vi "ELVIS III v1.0 Unreserve UART.vi"(8 "error in (no error)":errorcluster, 10 "VISA resource name in":refnum<visa-resource-name>, 11 "myRIO FPGA Ref In":T1) -> (0 "error out":errorcluster)   [LabVIEW 2021]
uses:
  <vilib>/myRIO/Common/Instrument Driver Framework/Utilities/typedefs/Generic FPGA Reference.ctl
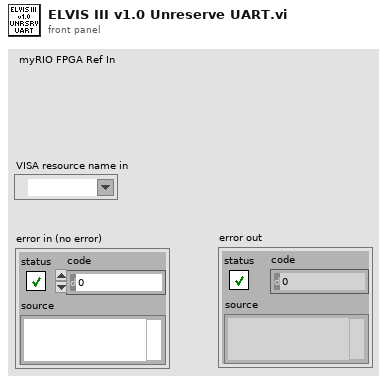
[diagram p1: front panel]
types:
  T1 = typedef "Generic FPGA Reference.ctl" = refnum<k20>
  T2 = typedef "ELVIS III v1.0 Channel Reservation List.ctl" = T3[]
  T3 = typedef "ELVIS III v1.0 Channel Reservation Info.ctl" = cluster{"Channel Name":string, "Connector":T4, "MutexIDs":u32[]}
  T4 = typedef "ELVIS III v1.0 Connector List.ctl" = enum32{"None", "ConnectorA", "ConnectorB"}
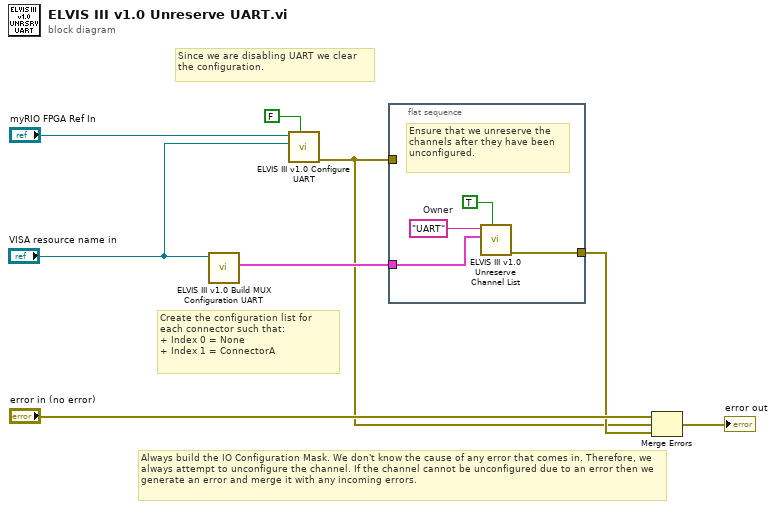
[diagram p0: block diagram]
diagram:
  # "Since we are disabling UART we clear the configuration."
  # "Always build the IO Configuration Mask. We don't know the cause of any error that comes in. Therefore, we always attempt to unconfigure the channel. If the channel cannot be unconfigured due to an error then we generate an error and merge it with any incoming errors."
  # "Create the configuration list for each connector such that:\n+ Index 0 = None\n+ Index 1 = ConnectorA"
  n1 = call <vilib>:"ELVIS III v1.0 Build MUX Configuration UART.vi"("VISA resource name in"="VISA resource name in") -> ("Channel Reservation List"=w6:T2)  [unwired: 10 in]
  n2 = call <vilib>:"ELVIS III v1.0 Configure UART.vi"("Reserve?"=FALSE ("Clear?"), "VISA resource name in"="VISA resource name in", "myRIO FPGA Ref"="myRIO FPGA Ref In") -> ("error out"=w1:errorcluster)  [unwired: 8 in]
  n3 = flat-sequence {
    tunnel: w6 -> [w11]
    tunnel: [w10] -> w2
    tunnel: w1 -> [_]
    frame #0 {
      w12 = "UART"  # Owner
      # "Ensure that we unreserve the channels after they have been unconfigured."
      n4 = call <vilib>:"ELVIS III v1.0 Unreserve Channel List.vi"("Allow multiple opens?"=TRUE, "Channel Reservation List"=w11, "Owner"=w12) -> ("error out"=w10:errorcluster)  [unwired: 8 in]
    }
  }
  n5 = Merge Errors("error in (no error)", w1, w2) -> (→"error out":errorcluster)
